vi "Start Block Cycle.vi"(9 "Block IO Control":T1={"Skip Next Read"=FALSE, "Skip Write"=FALSE, "Read Timeout"=-1}, 10 "i":i32, 11 "Worker Block In":T2={"Block Status"=refnum, "Command Queue"=refnum, "Status"={"Block Status"={"State"=enum."Init", "Next State"=enum."Idle", "Runs"=0, "i"=0, "Init"=FALSE, "Started"=FALSE, "Closing"=FALSE, "Step"=FALSE, "Phase"=enum."N/A", "Worker"=""}, "Error"={"status"=FALSE, "code"=0, "source"=""}}}) -> (1 "Read Timeout":i32, 3 "Worker Block":T2={"Block Status"=refnum, "Command Queue"=refnum, "Status"={"Block Status"={"State"=enum."Init", "Next State"=enum."Idle", "Runs"=0, "i"=0, "Init"=FALSE, "Started"=FALSE, "Closing"=FALSE, "Step"=FALSE, "Phase"=enum."N/A", "Worker"=""}, "Error"={"status"=FALSE, "code"=0, "source"=""}}}, 4 "Do Read":bool, 6 "Close":bool)   [LabVIEW 2022 SP3, in "FlexBlocks Support.lvlib"]
uses:
  FlexBlocks Support.lvlib
  Worker Block.ctl
  Block Status with Error.ctl
  Block Status.ctl
  Block State.ctl
  Block Phase.ctl
  Block Command.ctl
  Block IO Control.ctl
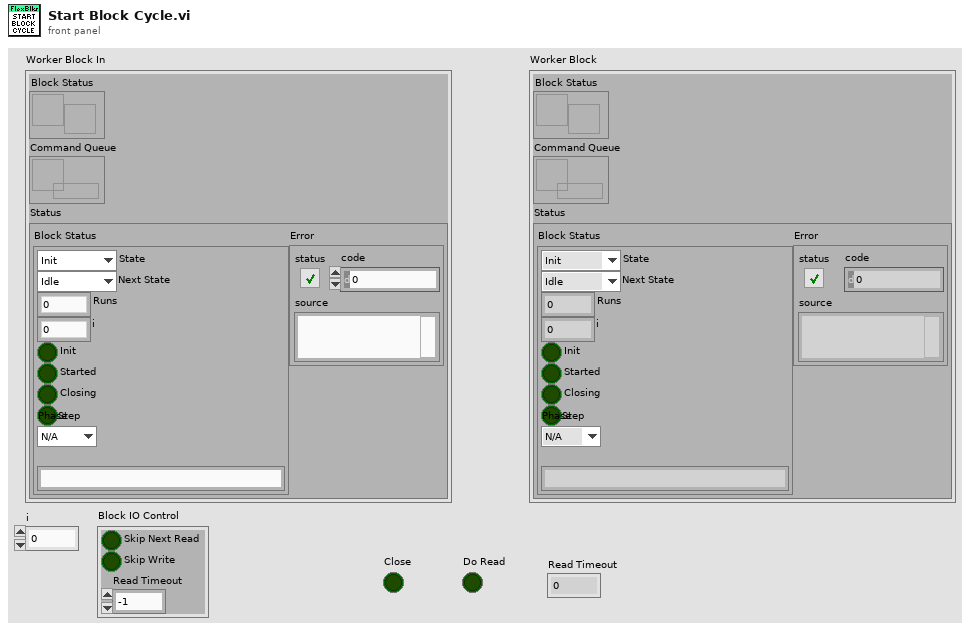
[diagram p1: front panel]
types:
  T1 = typedef "FlexBlocks Support.lvlib/Block IO Control.ctl" = cluster{"Skip Next Read":bool, "Skip Write":bool, "Read Timeout":i32}
  T2 = typedef "FlexBlocks Support.lvlib/Worker Block.ctl" = cluster{"Block Status":refnum<user-event>, "Command Queue":refnum<queue>, "Status":T3}
  T3 = typedef "FlexBlocks Support.lvlib/Block Status with Error.ctl" = cluster{"Block Status":T4, "Error":errorcluster}
  T4 = typedef "FlexBlocks Support.lvlib/Block Status.ctl" = cluster{"State":T5, "Next State":T5, "Runs":u32, "i":i32, "Init":bool, "Started":bool, "Closing":bool, "Step":bool, "Phase":T6, "Worker":string}
  T5 = typedef "FlexBlocks Support.lvlib/Block State.ctl" = enum16{"Idle", "Init", "Start", "Run", "Stop", "Close"}
  T6 = typedef "FlexBlocks Support.lvlib/Block Phase.ctl" = enum16{"N/A", "Read", "Work", "Write"}
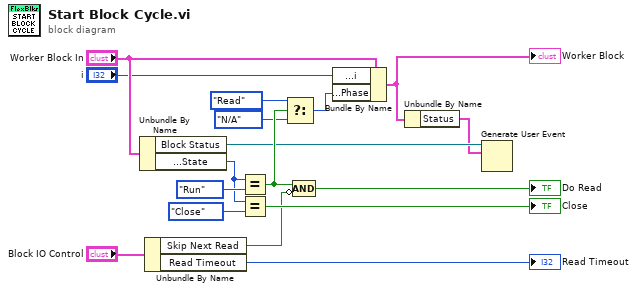
[diagram p0: block diagram]
diagram:
  n1 = Unbundle By Name("Worker Block In") -> ("Block Status"=w10:refnum<user-event>, "Status.Block Status.State"=w6:T5)
  n2 = Unbundle By Name("Block IO Control") -> ("Skip Next Read"=w1:bool, "Read Timeout"=→"Read Timeout":i32)
  n3 = Equal?(x=w6, y=Block_State."Run") -> (x = y?=w14:bool)
  n4 = Equal?(x=w6, y=Block_State."Close") -> (x = y?=→"Close":bool)
  n5 = Select(t=Block_Phase."Read" ("Status.Block Status.Phase"), s=w14, f=Block_Phase."N/A" ("Status.Block Status.Phase")) -> (s? t:f=w11:T6)
  n6 = Compound Arithmetic op=AND(w14, invert w1) -> (→"Do Read":bool)
  n7 = Bundle By Name(cluster="Worker Block In", "Status.Block Status.i"="i", "Status.Block Status.Phase"=w11) -> (w8:T2)
  "Worker Block" <- w8
  n8 = Unbundle By Name(w8) -> ("Status"=w9:T3)
  n9 = Generate User Event(user event=w10, event data cluster=w9) -> ()  [unwired: 2 in, 2 out]
